vi "DetectAnalyser.vi"(8 "error in (no error)":errorcluster, 11 "Microscope in":refnum<class "Microscope.lvclass">) -> (0 "error out":errorcluster, 3 "Microscope out":refnum<class "Microscope.lvclass">)   [LabVIEW 2020, in "Microscope.lvlib" / "Microscope.lvclass"]
uses:
  Microscope.lvclass
  Logic Layer/QuickNote/QuickNote/QuickNote.lvclass
  E:/Development/DevHardSoftware/MicroscopyFramework/Analyser/Analyser/Analyser.lvclass
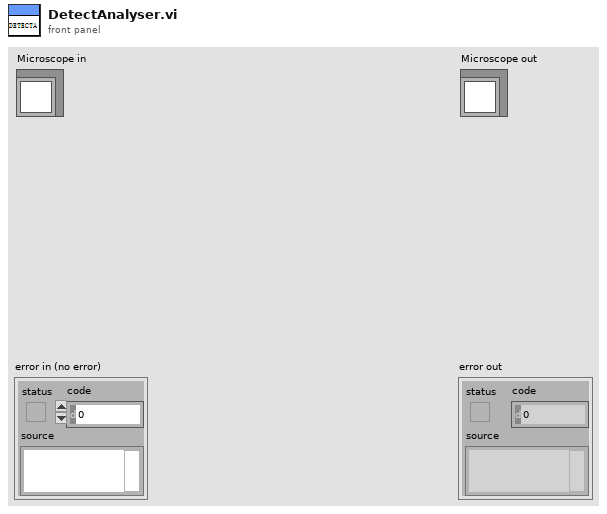
[diagram p1: front panel]
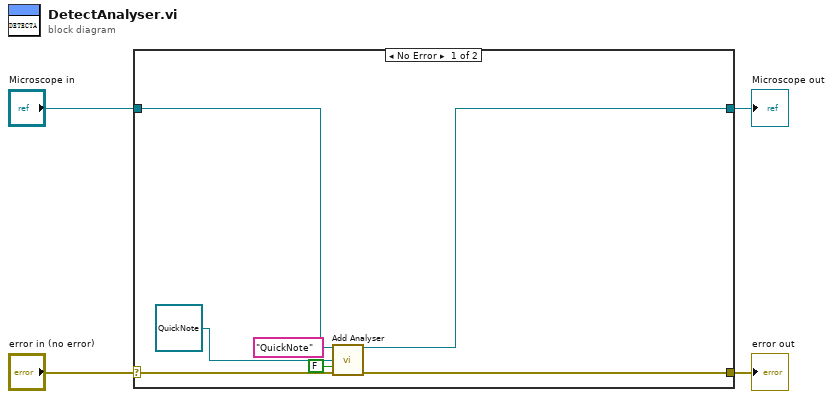
[diagram p0: block diagram]
diagram:
  n1 = case shown="No Error" "error in (no error)" {
    selector: "error in (no error)" -> [w11 w13]
    tunnel: [w10 w13] -> w3
    tunnel: [w8 w12] -> w1
    tunnel: "Microscope in" -> [w9 w12]
    frame No Error {
      n2 = call-dynamic "Add Analyser.vi"("Microscope in"=w9, "Label"="QuickNote", "Analyser"=refnum<class "QuickNote.lvclass"> refnum ("QuickNote.lvlib:QuickNote.lvclass"), "RegisterInPipleline?(F)"=FALSE, "error in (no error)"=w11) -> ("Microscope out"=w8:refnum<class "Microscope.lvclass">, "error out"=w10:errorcluster)  [unwired: 7 in, 2 out]
    }
    frame Error {
    }
  }
  "error out" <- w3
  "Microscope out" <- w1
